vi "WLAN_FrameAnalysis.vi"(8 "error in (no error)":errorcluster, 11 "input cluster":cluster{"t0":dbl, "dt":dbl, "Y":cdb[]}) -> (0 "error out":errorcluster, 1 "Constellation":cdb[](graph), 2 "Modulation parameter":T1, 3 "output bits":i8[](array[numeric]), 4 "Frequency offset":dbl, 5 "SIG valid?":bool, 6 "outputbitsHP":i8[](array[numeric]))   [LabVIEW 2022 SP3]
panel:
  out "size(s) 6":i32
  out "size(s) 5":i32
  out "size(s) 4":i32
  out "x+y":dbl
  out "Frequency offset(LTF)":dbl
  out "Frequency offset corrected signal 2":cluster{"t0":dbl, "dt":dbl, "Y":dbl[]}(graph)
  out "size(s) 3":i32
  out "size(s) 2":i32
  out "size(s)":i32
  out "Symbol numbers":i32
  out "encoded bit numbers":u32
  out "original bit numbers":u32
  out "Channel Esitimate":dbl[](graph)
  out "Frequency offset corrected signal":cluster{"t0":dbl, "dt":dbl, "Y":dbl[]}(graph)
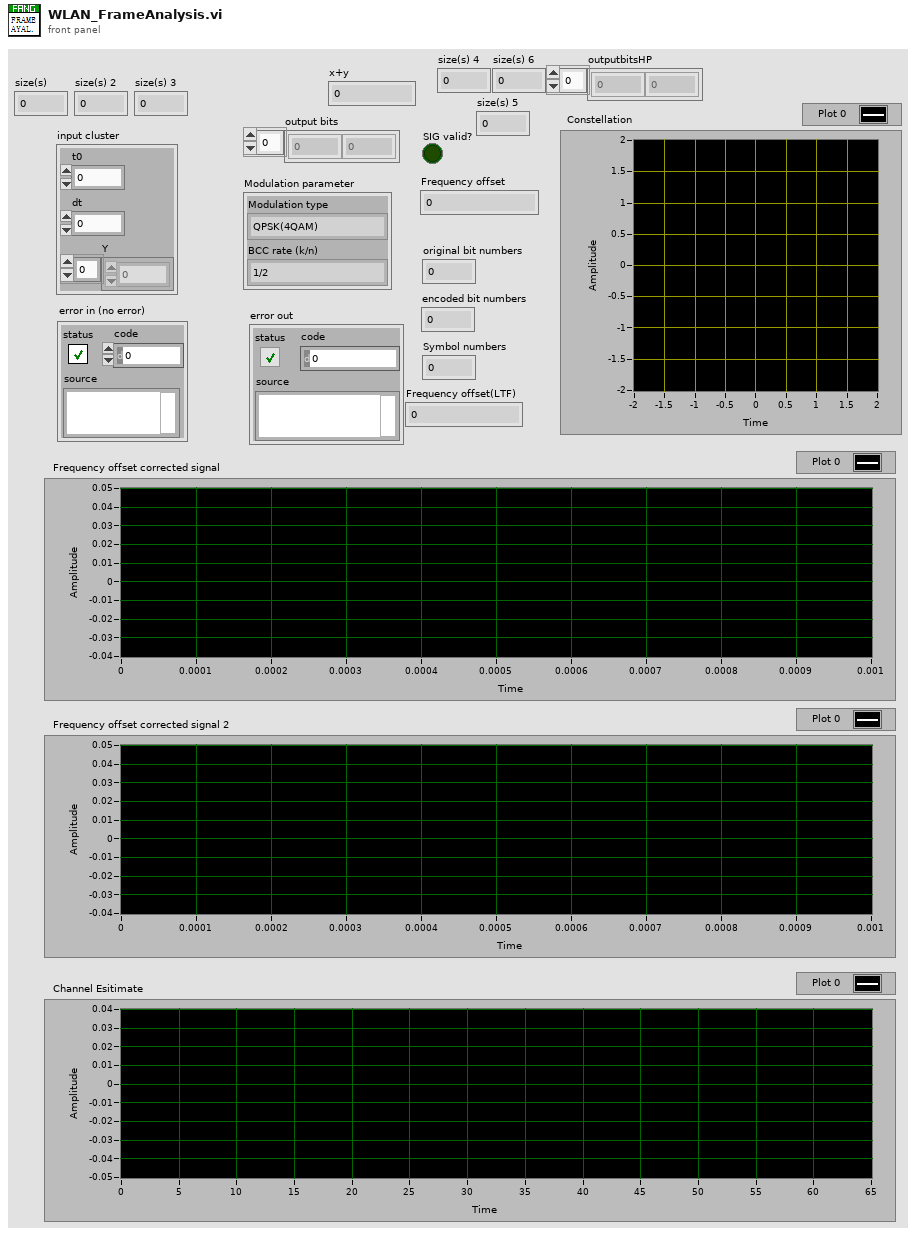
[diagram p1: front panel]
types:
  T1 = cluster{"Modulation type":enum16{"QPSK(4QAM)", "64QAM", "16QAM", "BPSK"}, "BCC rate (k/n)":enum16{"1/2", "2/3", "3/4"}}
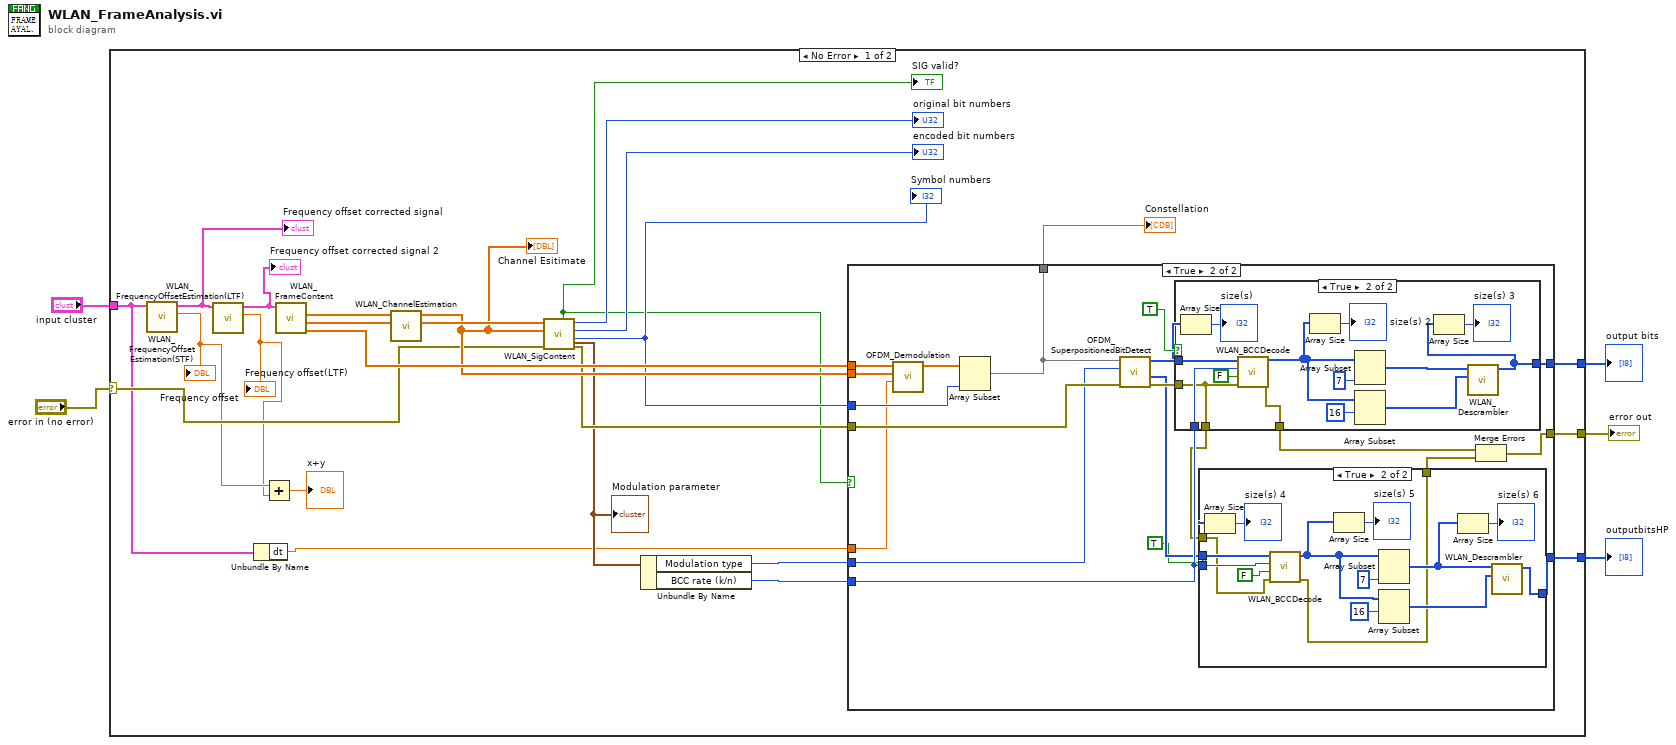
[diagram p0: block diagram]
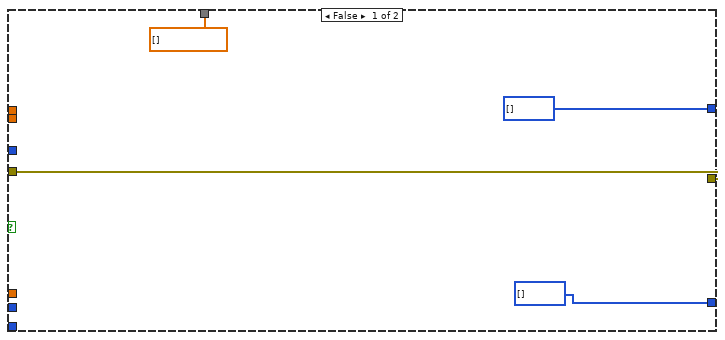
[diagram p2: hidden frame]
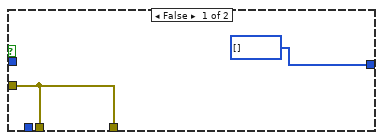
[diagram p3: hidden frame]
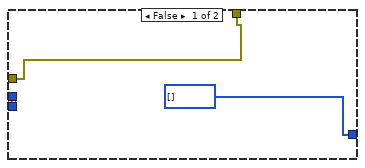
[diagram p4: hidden frame]
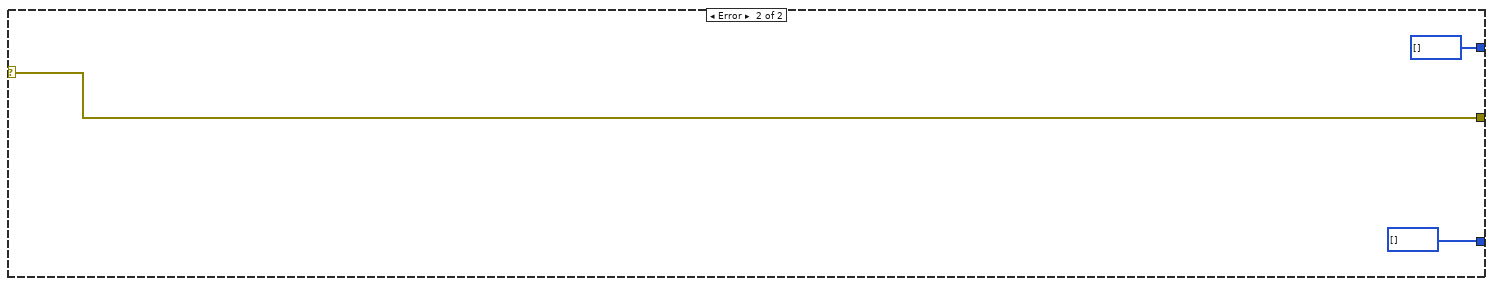
[diagram p5: hidden frame]
diagram:
  n1 = case shown="No Error" "error in (no error)" {
    selector: "error in (no error)" -> [w14 w87]
    tunnel: "input cluster" -> [w8 _]
    tunnel: [w21 w87] -> w4
    tunnel: [w20 i8[] [] ("scrambled bits")] -> w3
    tunnel: [w6 i8[] [] ("scrambled bits")] -> w1
    frame No Error {
      n2 = call "WLAN_FrequencyOffsetEstimation(STF).vi"("output cluster"=w8) -> ("Frequency offset(STF)"=w12:dbl, "output cluster 2"=w13:cluster{"t0":dbl, "dt":dbl, "Y":cdb[]})  [unwired: 8 in]
      "Frequency offset corrected signal" <- w13
      "Frequency offset" <- w12
      n3 = call "WLAN_FrequencyOffsetEstimation(LTF).vi"("input cluster"=w13) -> ("Frequency offset(LTF)"=w11:dbl, "output cluster"=w9:cluster{"t0":dbl, "dt":dbl, "Y":cdb[]})  [unwired: 9 in]
      "Frequency offset corrected signal 2" <- w9
      "Frequency offset(LTF)" <- w11
      n4 = Unbundle By Name(w8) -> ("dt"=w7:dbl)
      n5 = Add(x=w12, y=w11) -> (x+y=→"x+y":dbl)
      n6 = call "WLAN_FrameContent.vi"("Input cluster"=w9) -> ("DATA"=w29:cdb[], "SIG"=w27:cdb[], "LTF"=w28:cdb[])  [unwired: 7 in, 1 out]
      n7 = call "WLAN_ChannelEstimation.vi"("LTF"=w28) -> ("Frequency estimation"=w26:cdb[])  [unwired: 10 in]
      "Channel Esitimate" <- w26
      n8 = call "WLAN_SigContent.vi"("error in (no error)"=w14, "Frequency channel estimation"=w26, "SIG"=w27) -> ("error out"=w25:errorcluster, "Symbol numbers"=w22:i32, "encoded bit numbers"=→"encoded bit numbers":u32, "original bit numbers"=→"original bit numbers":u32, "Modulation parameter"=w19:T1, "SIG valid?"=w15:bool)  [unwired: 3 in]
      "Modulation parameter" <- w19
      "Symbol numbers" <- w22
      "SIG valid?" <- w15
      n9 = Unbundle By Name(w19) -> ("Modulation type"=w18:enum16{"QPSK(4QAM)", "64QAM", "16QAM", "BPSK"}, "BCC rate (k/n)"=w17:enum16{"1/2", "2/3", "3/4"})
      n10 = case shown="True" w15 {
        tunnel: w29 -> [_ w53]
        tunnel: [w33 w34] -> w21
        tunnel: w26 -> [_ w51]
        tunnel: w25 -> [w33 w50]
        tunnel: w22 -> [_ w49]
        tunnel: w18 -> [_ w48]
        tunnel: [i8[] [] ("scrambled bits") w44] -> w20
        tunnel: w17 -> [_ w42]
        tunnel: [cdb[] [] w46] -> w16
        tunnel: w7 -> [_ w43]
        tunnel: [i8[] [] ("scrambled bits") w40] -> w6
        frame False {
        }
        frame True {
          n11 = call "OFDM_Demodulation.vi"("sampling period"=w43, "Frequency channel estimation"=w51, "Input sequence"=w53) -> ("Output sequence"=w52:cdb[])  [unwired: 8 in]
          n12 = Array Subset(array=w52, length=w49) -> (w46:cdb[])  [unwired: 1 in]
          n13 = call "OFDM_SuperpositionedBitDetect.vi"("Input symbols"=w46, "Modulation type"=w48, "error in (no error)"=w50) -> ("OutputbitsLP"=w45:i8[], "OutputbitsHP"=w41:i8[], "error out"=w47:errorcluster)  [unwired: 5 in]
          n14 = case shown="True" TRUE ("need add zeros?") {
            tunnel: w47 -> [w54 w56]
            tunnel: [w54 w69] -> w36
            tunnel: w45 -> [_ w63]
            tunnel: [i8[] [] ("scrambled bits") w58] -> w44
            tunnel: w42 -> [_ w57]
            tunnel: [w54 w56] -> w37
            frame False {
            }
            frame True {
              n15 = Array Size(array=w63) -> (size(s)=→"size(s)":i32)
              n16 = call "WLAN_BCCDecode.vi"("error in (no error)"=w56, "need add zeros?"=FALSE, "BCC rate (k/n)"=w57, "input bit stream"=w63) -> ("error out"=w69:errorcluster, "output bit stream"=w60:i8[])  [unwired: 6 in]
              n17 = Array Size(array=w60) -> (size(s)=→"size(s) 2":i32)
              n18 = Array Subset(array=w60, length=7) -> (w65:i8[])  [unwired: 1 in]
              n19 = Array Subset(array=w60, index=16) -> (w66:i8[])  [unwired: 1 in]
              n20 = call "WLAN_Descrambler.vi"("scrambler initial bits"=w65, "data bits"=w66) -> ("scrambled bits"=w58:i8[])  [unwired: 7 in]
              n21 = Array Size(array=w58) -> (size(s)=→"size(s) 3":i32)
            }
          }
          n22 = case shown="True" TRUE ("need add zeros?") {
            tunnel: w42 -> [_ w84]
            tunnel: w41 -> [_ w83]
            tunnel: [i8[] [] ("scrambled bits") w76] -> w40
            tunnel: w37 -> [w70 w73]
            tunnel: [w70 w72] -> w35
            frame False {
            }
            frame True {
              n23 = Array Size(array=w83) -> (size(s)=→"size(s) 4":i32)
              n24 = call "WLAN_BCCDecode.vi"("error in (no error)"=w73, "need add zeros?"=FALSE, "BCC rate (k/n)"=w84, "input bit stream"=w83) -> ("error out"=w72:errorcluster, "output bit stream"=w80:i8[])  [unwired: 6 in]
              n25 = Array Size(array=w80) -> (size(s)=→"size(s) 5":i32)
              n26 = Array Subset(array=w80, length=7) -> (w75:i8[])  [unwired: 1 in]
              n27 = Array Subset(array=w80, index=16) -> (w77:i8[])  [unwired: 1 in]
              n28 = Array Size(array=w75) -> (size(s)=→"size(s) 6":i32)
              n29 = call "WLAN_Descrambler.vi"("scrambler initial bits"=w75, "data bits"=w77) -> ("scrambled bits"=w76:i8[])  [unwired: 7 in]
            }
          }
          n30 = Merge Errors(w36, w35) -> (w34:errorcluster)
        }
      }
      "Constellation" <- w16
    }
    frame Error {
    }
  }
  "error out" <- w4
  "output bits" <- w3
  "outputbitsHP" <- w1
